vi "利用SQL语句访问数据库.vi"(0 "connection reference":T1, 1 "数据库名称":string, 2 "TABLE":string, 3 "模拟运行":bool, 4 "数据库操作":enum16{"SELECT", "UPDATE", "INSERT", "DELETE"}(ring)=enum."DELETE", 5 "error in (no error)":errorcluster, 6 "附件条件":bool, 7 "附加语句":string, 8 "one column data":string[](array[string]), 9 "Insert Data":string[](array[string])=["5", "D", "5", "2015/1/19 14:41:15"], 10 "待操作的列名":string, 11 "待操作的列名对应的数据":string, 13 "columns":string[](array[string])) -> (14 "connection reference 2":T1, 18 "数据":string[][](array[string]), 19 "error out":errorcluster)   [LabVIEW 2018]
uses:
  <vilib>/addons/database/Connection.llb/Conn ObjectReference.ctl
  <vilib>/addons/database/Connection.llb/DB Tools Open Connec (String).vi
  <vilib>/addons/database/Connection.llb/Conn Execute.vi
  <vilib>/addons/database/Recordset.llb/Rec Fetch Recordset Data (R).vi
  <vilib>/addons/database/Recordset.llb/Rec Destroy - Connection.vi
  <vilib>/addons/database/NI_Database_API.lvlib
panel:
  # "UPDATE"
  # "one column data:\n                        列名1\n                        列名1数据\n                        需要操作的列的列名\n                         需要操作的列的数据"
  # "SELECT"
  # "DELETE"
  # "主键不能用单引号,更新多个数据\n时，在第一项中输入列名1='',\n列名2='',......列名n，第二项中输入\n列名n对应的数据"
  # "INSERT"
  # "两者数组大小必须保持一样的"
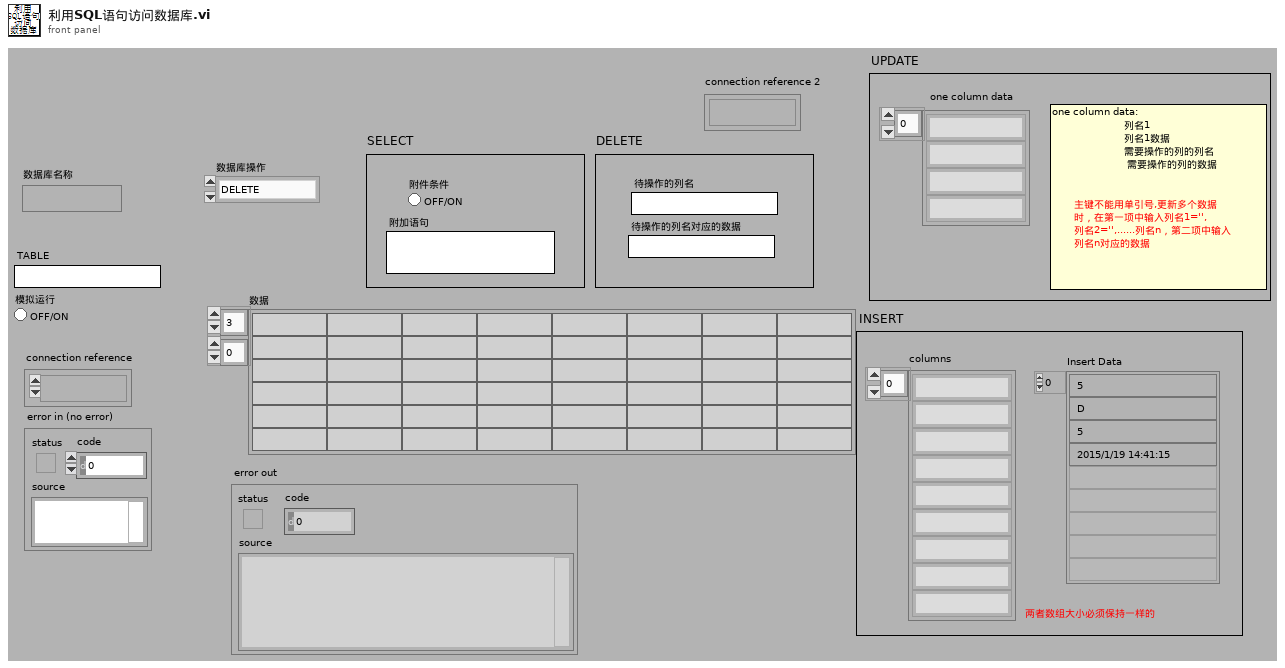
[diagram p1: front panel]
types:
  T1 = typedef "NI_Database_API.lvlib/Conn ObjectReference.ctl" = refnum<k1>
  T2 = typedef "NI_Database_API.lvlib/Rec ObjectReference.ctl" = refnum<k1>
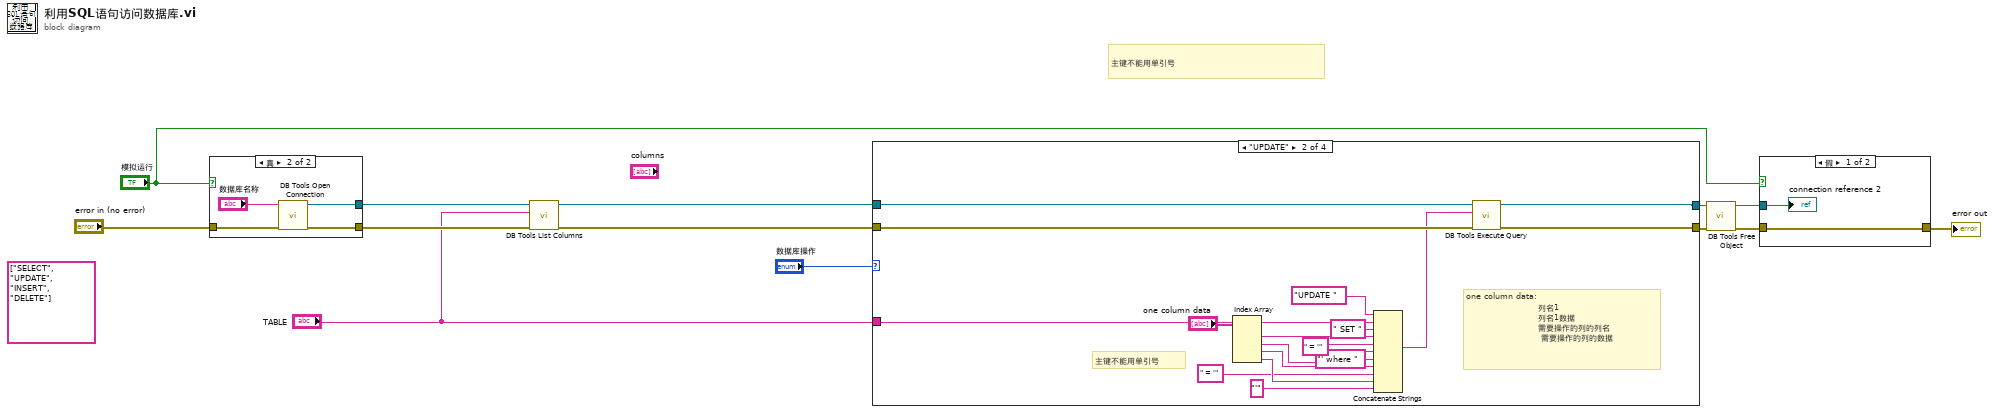
[diagram p0: block diagram]
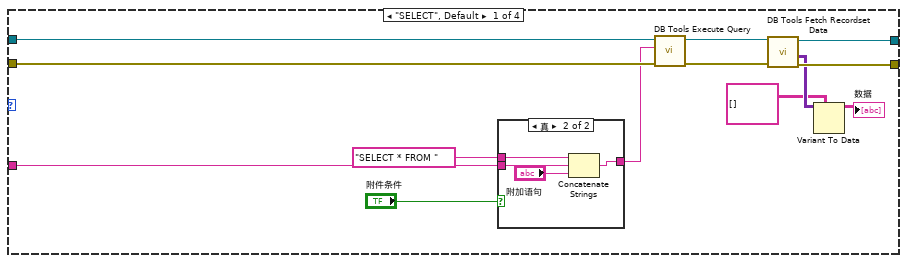
[diagram p2: hidden frame]
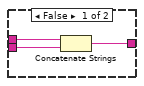
[diagram p3: hidden frame]
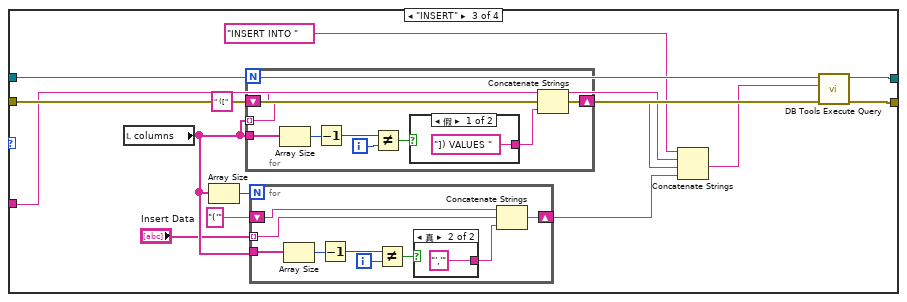
[diagram p4: hidden frame]
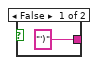
[diagram p5: hidden frame]
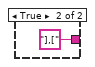
[diagram p6: hidden frame]
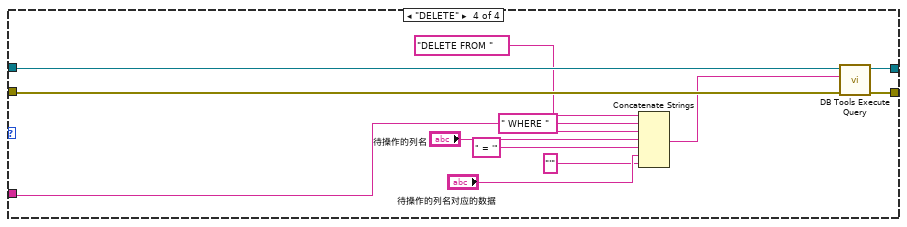
[diagram p7: hidden frame]
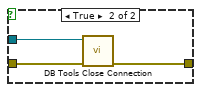
[diagram p8: hidden frame]
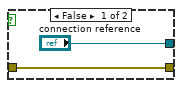
[diagram p9: hidden frame]
diagram:
  (unwired) string[] ["SELECT", "UPDATE", "INSERT", "DELETE"]
  # "主键不能用单引号"
  n1 = case shown="真" "模拟运行" {
    tunnel: ["connection reference" w19] -> w5
    tunnel: "error in (no error)" -> [w14 w17]
    tunnel: [w14 w16] -> w4
    frame False {
    }
    frame True {
      n2 = call-poly <vilib>:"DB Tools Open Connection.vi"("error in (no error)"=w17, "connection information"="数据库名称") -> ("error out"=w16:errorcluster, "connection reference"=w19:T1)  [unwired: 6 in]
    }
  }
  n3 = call <vilib>:"DB Tools List Columns.vi"("error in (no error)"=w4, "table"="TABLE", "connection reference"=w5) -> ("error out"=w1:errorcluster, "connection reference out"=w2:T1)  [unwired: 1 in, 2 out]
  n4 = case shown="\"UPDATE\"" "数据库操作" {
    tunnel: [w30 w43 w68 w104] -> w13
    tunnel: [w29 w42 w67 w103] -> w12
    tunnel: w2 -> [w28 w46 w70 w102]
    tunnel: w1 -> [w27 w45 w69 w101]
    tunnel: "TABLE" -> [w20 w54 w58 w99]
    frame "SELECT", Default {
      n5 = case shown="真" "附件条件" {
        tunnel: "SELECT * FROM " ("字符串") -> [w35 w39]
        tunnel: [w33 w37] -> w21
        tunnel: w20 -> [w34 w36]
        frame False {
          n6 = Concatenate Strings(w35, w34) -> (w33:string)
        }
        frame True {
          n7 = Concatenate Strings(w39, w36, "附加语句") -> (w37:string)
        }
      }
      n8 = call-poly <vilib>:"DB Tools Execute Query.vi"("error in (no error)"=w27, "SQL query"=w21, "connection reference"=w28) -> ("error out"=w31:errorcluster, "recordset reference"=w32:T2)  [unwired: 5 in]
      n9 = call-poly <vilib>:"DB Tools Fetch Recordset Data.vi"("error in (no error)"=w31, "recordset reference"=w32) -> ("error out"=w29:errorcluster, "recordset data"=w26:variant[][], "recordset reference out"=w30:T2)  [unwired: 3 in]
      n10 = Variant To Data(type=string[][] [], Variant=w26) -> (data=→"数据":string[][])  [unwired: 1 in, 1 out]
    }
    frame "UPDATE" {
      # "主键不能用单引号"
      # "one column data:\n                        列名1\n                        列名1数据\n                        需要操作的列的列名\n                         需要操作的列的数据"
      n11 = Index Array(array="one column data") -> (element #1=w52:string, element #2=w51:string, element #3=w49:string, element #4=w47:string)  [unwired: 4 in]
      n12 = Concatenate Strings("UPDATE ", w54, " SET " ("字符串"), w52, " = '" ("字符串"), w51, "' where " ("字符串"), w49, " = '" ("字符串"), w47, "'" ("字符串")) -> (w44:string)
      n13 = call-poly <vilib>:"DB Tools Execute Query.vi"("error in (no error)"=w45, "SQL query"=w44, "connection reference"=w46) -> ("error out"=w42:errorcluster, "recordset reference"=w43:T2)  [unwired: 5 in]
    }
    frame "INSERT" {
      n14 = local read "columns"() -> (w65:string[])
      n15 = Array Size(array=w65) -> (size(s)=w64:i32)
      n16 = for {
        tunnel: w65 -> [w90] mode=indexing
        shift-right: [w89] -> w62
        shift-left: " ([" -> [w88]
        tunnel: w65 -> [w86]
        i -> [w83]
        n17 = Array Size(array=w86) -> (size(s)=w85:i32)
        n18 = Decrement(x=w85) -> (x-1=w84:i32)
        n19 = Not Equal?(x=w84, y=w83) -> (x != y?=w82:bool)
        n20 = case shown="假" w82 {
          tunnel: ["]) VALUES " ("字符串") "],[" ("字符串")] -> w87
          frame False {
          }
          frame True {
          }
        }
        n21 = Concatenate Strings(w88, w90, w87) -> (w89:string)
      }
      n22 = for {
        N: w64 -> [_]
        tunnel: "Insert Data" -> [w79] mode=indexing
        shift-right: [w78] -> w63
        shift-left: "('" -> [w77]
        tunnel: w65 -> [w75]
        i -> [w72]
        n23 = Array Size(array=w75) -> (size(s)=w74:i32)
        n24 = Decrement(x=w74) -> (x-1=w73:i32)
        n25 = Not Equal?(x=w73, y=w72) -> (x != y?=w71:bool)
        n26 = case shown="真" w71 {
          tunnel: ["')" ("字符串") "','" ("字符串")] -> w76
          frame False {
          }
          frame True {
          }
        }
        n27 = Concatenate Strings(w77, w79, w76) -> (w78:string)
      }
      n28 = Concatenate Strings("INSERT INTO ", w58, w62, w63) -> (w57:string)
      n29 = call-poly <vilib>:"DB Tools Execute Query.vi"("error in (no error)"=w69, "SQL query"=w57, "connection reference"=w70) -> ("error out"=w67:errorcluster, "recordset reference"=w68:T2)  [unwired: 5 in]
    }
    frame "DELETE" {
      n30 = Concatenate Strings("DELETE FROM " ("字符串"), w99, " WHERE " ("字符串"), "待操作的列名", " = '" ("字符串"), "待操作的列名对应的数据", "'" ("字符串")) -> (w94:string)
      n31 = call-poly <vilib>:"DB Tools Execute Query.vi"("error in (no error)"=w101, "SQL query"=w94, "connection reference"=w102) -> ("error out"=w103:errorcluster, "recordset reference"=w104:T2)  [unwired: 5 in]
    }
  }
  n32 = call-poly <vilib>:"DB Tools Free Object.vi"("error in (no error)"=w12, "recordset reference"=w13) -> ("error out"=w8:errorcluster, "connection reference"=w11:T1)  [unwired: 8 in]
  n33 = case shown="假" "模拟运行" {
    tunnel: w11 -> [w106 w109]
    tunnel: w8 -> [w105 w108]
    tunnel: [w105 w107] -> w7
    frame False {
      "connection reference 2" <- w106
    }
    frame True {
      n34 = call <vilib>:"DB Tools Close Connection.vi"("error in (no error)"=w108, "connection reference"=w109) -> ("error out"=w107:errorcluster)  [unwired: 5 in]
    }
  }
  "error out" <- w7
